vi "poly_asynch_wait_notify.vi"(8 "error in":errorcluster, 10 "asynch wait ref in":T1) -> (0 "error out":errorcluster)   [LabVIEW 2015]
uses:
  cores/asynch_wait_ref.ctl
  cores/boolean_notifier.ctl
  poly_notify_boolean_notifier_notifier.vi
  poly_timing_tools_eco_plus.vi
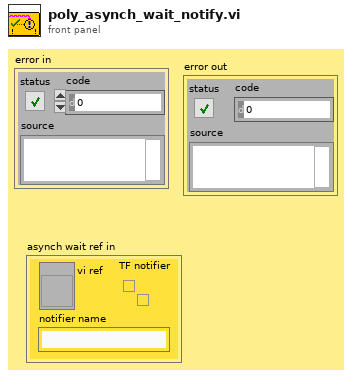
[diagram p1: front panel]
types:
  T1 = typedef "asynch_wait_ref.ctl" = cluster{"vi ref":refnum<vi>, "TF notifier":T2, "notifier name":string}
  T2 = typedef "boolean_notifier.ctl" = refnum<notifier>
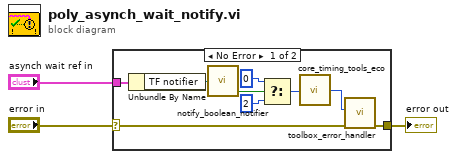
[diagram p0: block diagram]
diagram:
  n1 = case shown="No Error" "error in" {
    selector: "error in" -> [w9 w13]
    tunnel: [w8 w13] -> w3
    tunnel: "asynch wait ref in" -> [w12 _]
    frame No Error {
      n2 = Unbundle By Name(w12) -> ("TF notifier"=w5:T2)
      n3 = call-poly "notify_boolean_notifier.vi"("TF notifier"=w5) -> ("notified?"=w4:bool)  [unwired: 8 in]
      n4 = Select(t=0 ("code (0 = no error)"), s=w4, f=2) -> (s? t:f=w7:i32)
      n5 = call-poly "core_timing_tools_eco.vi"("code (w/out eco)"=w7) -> ("code (+ eco)"=w6:i32)  [unwired: 4 in]
      n6 = call "toolbox_error_handler.vi"("error in (no error)"=w9, "code (0 = no error)"=w6) -> ("error out"=w8:errorcluster)  [unwired: 8 in, 1 out]
    }
    frame Error {
    }
  }
  "error out" <- w3
